vi "SavedSettingsAsStringArray.vi"(8 "error in (no error)":errorcluster, 10 "Tag":string, 11 "SavedSettings in":refnum<vi>) -> (0 "error out":errorcluster, 2 "Selection":string[](array[string]), 3 "SavedSettings out":refnum<vi>)   [LabVIEW 2021]
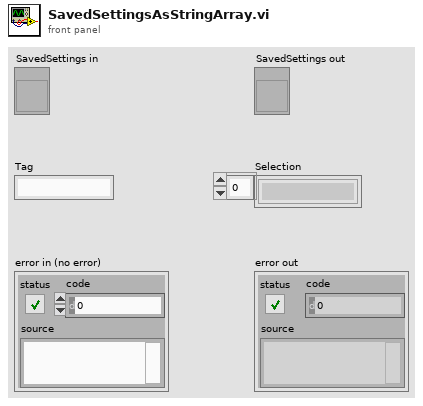
[diagram p1: front panel]
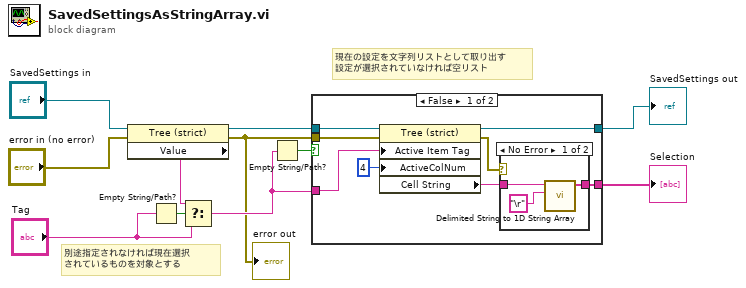
[diagram p0: block diagram]
diagram:
  # "別途指定されなければ現在選択\nされているものを対象とする"
  # "現在の設定を文字列リストとして取り出す\n設定が選択されていなければ空リスト"
  n1 = property class="Tree (strict)"(reference="SavedSettings in", error in="error in (no error)") -> (reference out=w7:refnum<vi>, error out=w1:errorcluster, "Value"=w4:string)
  "error out" <- w1
  n2 = Empty String/Path?(string/path="Tag") -> (empty?=w5:bool)
  n3 = Select(t=w4, s=w5, f="Tag") -> (s? t:f=w3:string)
  n4 = Empty String/Path?(string/path=w3) -> (empty?=w8:bool)
  n5 = case shown="False" w8 {
    tunnel: w7 -> [w17 w23]
    tunnel: w3 -> [w19 _]
    tunnel: [w14 _] -> w11
    tunnel: w1 -> [w13 _]
    tunnel: [w16 w23] -> w6
    frame False {
      n6 = property class="Tree (strict)"(reference=w17, error in=w13, "Active Item Tag"=w19, "ActiveColNum"=4 ("Active Cell:Active Column Number")) -> (reference out=w16:refnum<vi>, error out=w12:errorcluster, "Cell String"=w15:string)
      n7 = case shown="No Error" w12 {
        tunnel: w15 -> [w21 _]
        tunnel: [w20 _] -> w14
        frame No Error {
          n8 = call <vilib>:"Delimited String to 1D String Array.vi"("delimiter"="\r", "delimited string"=w21) -> ("string array"=w20:string[])  [unwired: 9 in]
        }
        frame Error {
        }
      }
    }
    frame True {
    }
  }
  "Selection" <- w11
  "SavedSettings out" <- w6
